vi "Configure 5752 Module (FPGA).vi"() -> (1 "IO Module Status":T1)   [LabVIEW 2012]
uses:
  <vilib>/rvi/eio/common/nirviEmuTemplateMethod_errors.vi
  <vilib>/eio/EIONode/EIONode.xnode
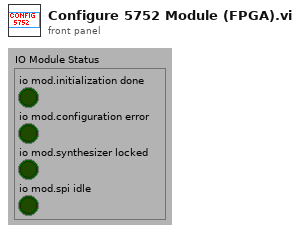
[diagram p1: front panel]
types:
  T1 = cluster{"io mod.initialization done":bool, "io mod.configuration error":bool, "io mod.synthesizer locked":bool, "io mod.spi idle":bool}
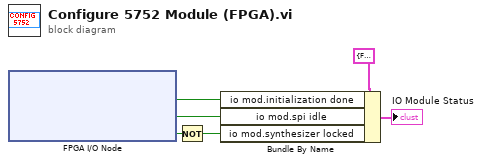
[diagram p0: block diagram]
diagram:
  n1 = xnode "FPGA I/O Node"() -> ("IO Module\\InitDone"=w5:bool, "IO Module\\cSpiIdle"=w4:bool, "IO Module\\PllUnlocked"=w3:bool)  [unwired: 3 in, 3 out]
  n2 = Not(x=w3) -> (.not. x?=w1:bool)
  n3 = Bundle By Name(cluster=T1 {"io mod.initialization done"=FALSE, "io mod.configuration error"=FALSE, "io mod.synthesizer locked"=FALSE, "io mod.spi idle"=FALSE} ("IO Module Status"), "io mod.initialization done"=w5, "io mod.spi idle"=w4, "io mod.synthesizer locked"=w1) -> (→"IO Module Status":T1)
